vi "Auton Gyro Drive.vi"(9 "Heading target":dbl, 10 "Y Speed":dbl, 11 "X Speed":dbl) -> ()   [LabVIEW 2014]
uses:
  Drivetrain Code/Drivetrain Control.ctl
  Drivetrain Code/Drivetrain Mode.ctl
  Robot Global Data.vi
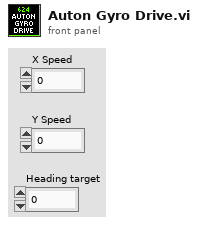
[diagram p1: front panel]
types:
  T1 = typedef "Drivetrain Mode.ctl" = enum16{"Manual", "Gyro Steer", "Vision Steer", "Drive Distance"}
  T2 = typedef "Drivetrain Control.ctl" = cluster{"Mode":T1, "Steer":dbl, "Y":dbl, "Heading Target":dbl, "Strafe X":dbl, "Y Target":dbl, "Strafe Target":dbl}
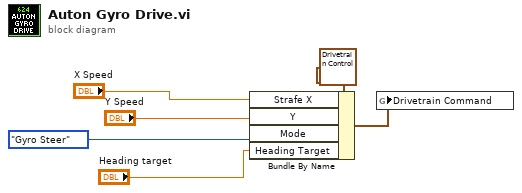
[diagram p0: block diagram]
diagram:
  n1 = Bundle By Name(cluster=T2 {"Mode"=enum."Gyro Steer", "Steer"=0.0, "Y"=0.0, "Heading Target"=0.0, "Strafe X"=0.0, "Y Target"=0.0, "Strafe Target"=0.0} ("Drivetrain Command"), "Strafe X"="X Speed", "Y"="Y Speed", "Mode"=Drivetrain_Mode."Gyro Steer", "Heading Target"="Heading target") -> (w5:T2)
  n2 = global write "Robot Global Data.vi" "Drivetrain Command"(w5) -> ()
